vi "fgv_ctrl-ref.vi"(7 "cmd":enum16{"write", "read"}(ring), 8 "error in":errorcluster, 11 "ref":T1) -> (0 "error out":errorcluster, 3 "ref out":T1)   [LabVIEW 2019]
uses:
  Ctrl/control_ref.ctl
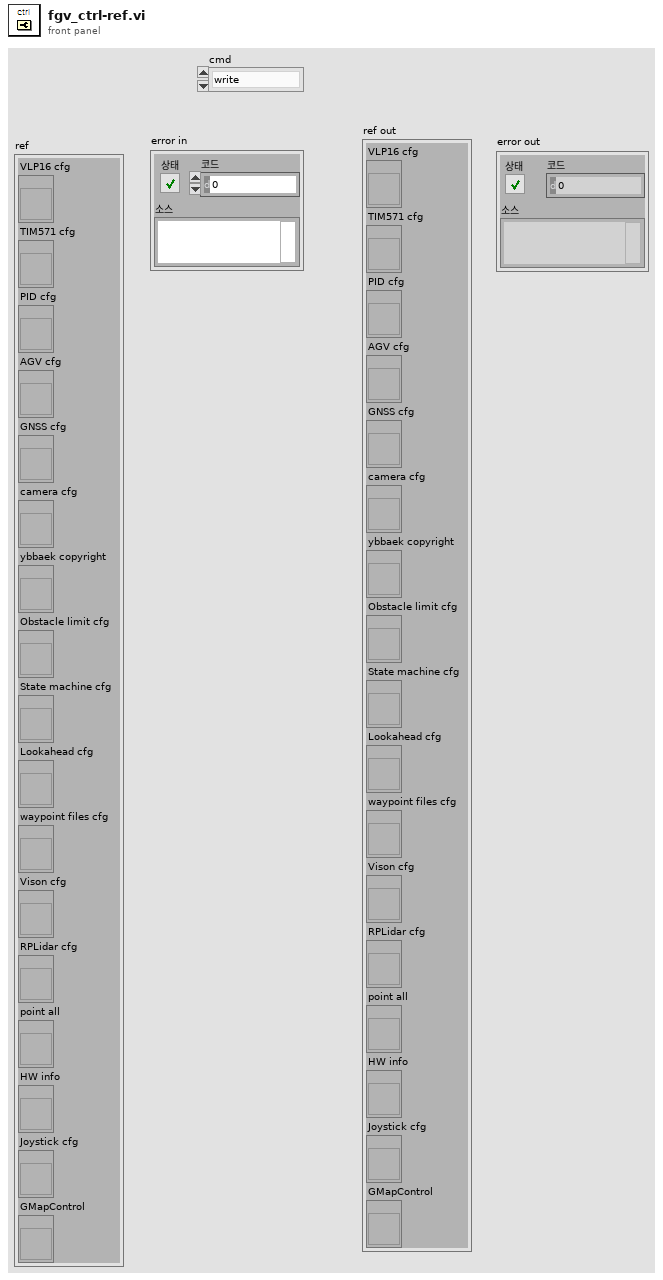
[diagram p1: front panel]
types:
  T1 = typedef "control_ref.ctl" = cluster{"VLP16 cfg":refnum<vi>, "TIM571 cfg":refnum<vi>, "PID cfg":refnum<vi>, "AGV cfg":refnum<vi>, "GNSS cfg":refnum<vi>, "camera cfg":refnum<vi>, "ybbaek copyright":refnum<vi>, "Obstacle limit cfg":refnum<vi>, "State machine cfg":refnum<vi>, "Lookahead cfg":refnum<vi>, "waypoint files cfg":refnum<vi>, "Vison cfg":refnum<vi>, "RPLidar cfg":refnum<vi>, "point all":refnum<vi>, "HW info":refnum<vi>, "Joystick cfg":refnum<vi>, "GMapControl":refnum<vi>}
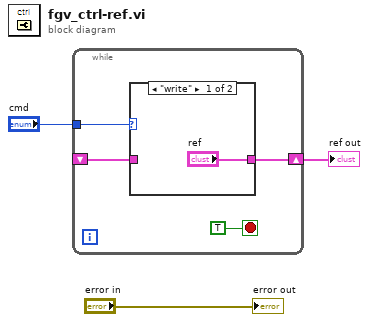
[diagram p0: block diagram]
diagram:
  n1 = while {
    tunnel: "cmd" -> [w6]
    shift-right: [w5] -> w1
    shift-left: _ -> [w4]
    stop <- TRUE stop-if-true
    n2 = case shown="\"write\"" w6 {
      tunnel: ["ref" w9] -> w5
      tunnel: w4 -> [_ w9]
      frame "write" {
      }
      frame "read", Default {
      }
    }
  }
  "ref out" <- w1
  "error out" <- "error in"
